vi "CASN_TRIM and HVDDL_TRIM Correction.vi"() -> ()   [LabVIEW 2010]
uses:
  Drivers/Telemetry/Typedef Command List.ctl
panel:
  out "error out":errorcluster
  out "Output":T1
  in  "error in (no error)":errorcluster
  in  "MICS Dongle Address":refnum<visa-resource-name>="COM5"
  in  "Input":T3={"Command"=enum."Get xPG Status", "Function"=enum."Open Session", "MICS_ID"=0, "EXID"=16773121, "Use Local"=TRUE, "Transceive Delay mS"=200.0, "CP_DATA IN"=[], "Parameters"=""} {"Transceive Delay mS" min=0.0 max=10000.0 step=1.0; "EXID" step=1 format="%.0x"; "MICS_ID" step=1 format="%06x"}
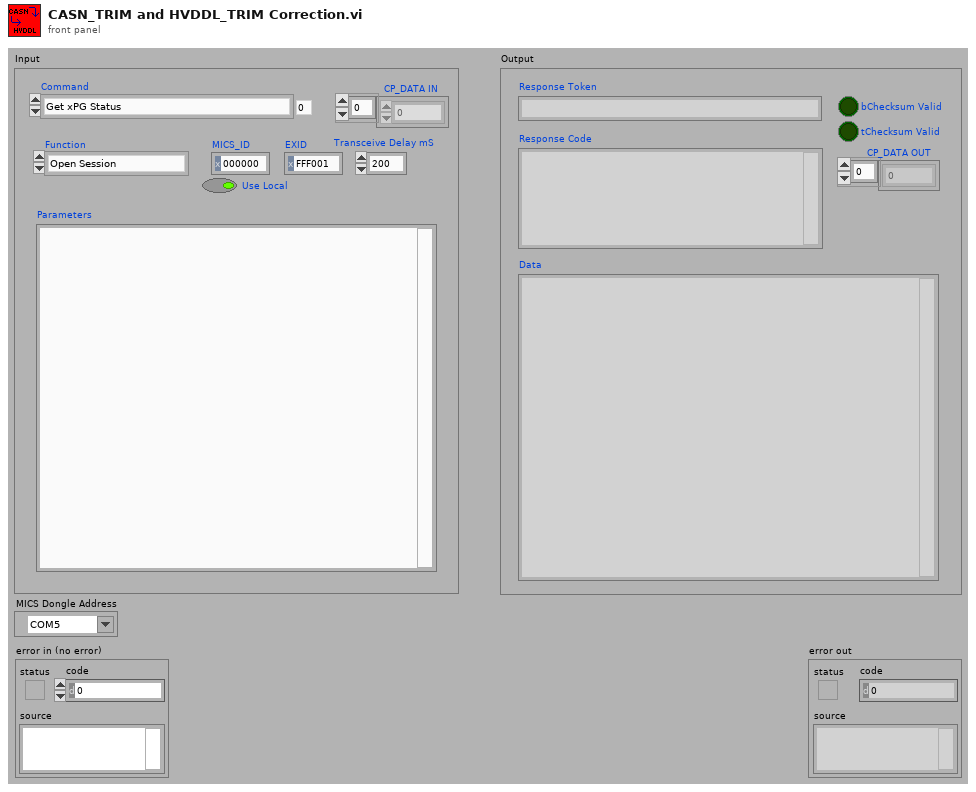
[diagram p1: front panel]
types:
  T1 = cluster{"Response Token":string, "Response Code":string, "bChecksum Valid":bool, "tChecksum Valid":bool, "CP_DATA OUT":u8[], "Data":string}
  T2 = typedef "Typedef Command List.ctl" = enum16{"Get xPG Status", "xPG Stimulation", "Select Program", "Increment Program Amplitude", "Decrement Program Amplitude", "Get PoP Constants", "Get PPC Constants", "Get Program Names", "Set Pulse Amplitude", "Increment Pulse Amplitude", "Decrement Pulse Amplitude", "Get Pulse Widths", "Set Pulse Widths", "Increment Pulse Width", "Decrement Pulse Width", "Get Program Frequency", "Set Program Frequency", "Increment Program Frequency", "Decrement Program Frequency", "Inject Event", "Charging Control", "Get xPG Identity", "Set xPG Identity", "Restore Program Defaults", "Get Program Definition", "Set Program Definition", "Get Program Constants", "Set Program Constants", "Get Configurable Device Parameters", "Set Configurable Device Parameters", "Get Pulse Constants", "Set Pulse Constants", "Get Lead Limits", "Set Lead Limits", "Get Channel Calibrations", "Set Channel Calibrations", "<reserved 2>", "<reserved 3>", "<reserved 4>", "<reserved 5>", "<reserved 6>", "<reserved 7>", "Get Stim Asic HV Calibrations", "Set Stim Asic HV Calibrations", "<reserved 8>", "<reserved 9>", "Get CP Data", "Set CP Data", "Clear Log", "Read Log", "Append Log", "Get Patient Program Runtime", "Set Patient Program Runtime", "Impedance Measurement", "Enter Storage Mode", "Echo Short", "Echo Long", "Get General Calibration", "Set General Calibration", "Get Trim List", "Set Trim List", "Get Counter", "Set Counter", "Get Test Stimulation", "Set Test Stimulation", "Get Titration Stimulation", "Set Titration Stimulation", "Get Ramp Time", "Set Ramp Time", "Get VBAT", "Set Software Description Block", "Get Software Description Block", "Write Memory", "Read Memory", "Reset xPG", "Erase Flash Block", "Write Vectors", "Read Vectors", "Diagnostic Data", "Set Background Impedance", "Get Background Impedence ", "Set Test Waveform", "Calibrate Channel", "Get Log Range", "Reserved 0x55", "Reserved 0x56", "MICS Options", "Pair PPC", "Pair POP", "Stop Bootloader", "Tune MICS", "MICS Diagnostics", "Undefined"}
  T3 = cluster{"Command":T2, "Function":enum16{"Open Session", "Close Session", "Downlink Only", "Uplink Only", "Transceive (DN -> UP)"}, "MICS_ID":u32, "EXID":u32, "Use Local":bool, "Transceive Delay mS":dbl, "CP_DATA IN":u8[], "Parameters":string}
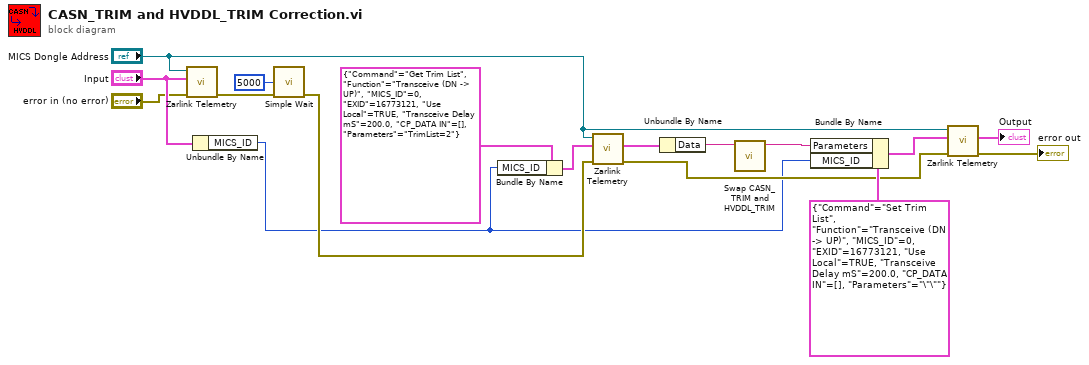
[diagram p0: block diagram]
diagram:
  n1 = call "Zarlink Telemetry.vi"("error in (no error)"="error in (no error)", "Input"="Input", "MICS Dongle Address"="MICS Dongle Address") -> ("error out"=w10:errorcluster)  [unwired: 6 in, 2 out]
  n2 = Unbundle By Name("Input") -> ("MICS_ID"=w4:u32)
  n3 = call "Simple Wait.vi"("mS"=u32 5000, "error in"=w10) -> ("error out"=w8:errorcluster)  [unwired: 12 in, 1 out]
  n4 = Bundle By Name(cluster=T3 {"Command"=enum."Get Trim List", "Function"=enum."Transceive (DN -> UP)", "MICS_ID"=0, "EXID"=16773121, "Use Local"=TRUE, "Transceive Delay mS"=200.0, "CP_DATA IN"=[], "Parameters"="TrimList=2"} ("Input"), "MICS_ID"=w4) -> (w5:T3)
  n5 = call "Zarlink Telemetry.vi"("error in (no error)"=w8, "Input"=w5, "MICS Dongle Address"="MICS Dongle Address") -> ("error out"=w11:errorcluster, "Output"=w16:T1)  [unwired: 6 in, 1 out]
  n6 = Unbundle By Name(w16) -> ("Data"=w17:string)
  n7 = call "Swap CASN_TRIM and HVDDL_TRIM.vi"("MICS DATA INITIAL"=w17) -> ("MICS DATA FINAL"=w14:string)  [unwired: 10 in]
  n8 = Bundle By Name(cluster=T3 {"Command"=enum."Set Trim List", "Function"=enum."Transceive (DN -> UP)", "MICS_ID"=0, "EXID"=16773121, "Use Local"=TRUE, "Transceive Delay mS"=200.0, "CP_DATA IN"=[], "Parameters"="\"\""} ("Input"), "Parameters"=w14, "MICS_ID"=w4) -> (w12:T3)
  n9 = call "Zarlink Telemetry.vi"("error in (no error)"=w11, "Input"=w12, "MICS Dongle Address"="MICS Dongle Address") -> ("error out"=→"error out":errorcluster, "Output"=→"Output":T1)  [unwired: 6 in, 1 out]
